vi "Autoscan_MirrorsToSPCM.vi"(6 "Device 4":refnum<k24>, 7 "reference":refnum<vi>, 9 "reference 3":refnum<vi>, 10 "reference 2":refnum<vi>, 11 ".NET Refnum in":refnum<k24>) -> (2 "Device":refnum<k24>, 3 ".NET Refnum out":refnum<k24>)   [LabVIEW 2023]
uses:
  C:/Users/nanometa/Documents/TCSPC_Git_Repo/Source/Thorlabs.MotionControl.FilterFlipperCLI.dll
  Thorlabs.MotionControl.FilterFlipperCLI.dll
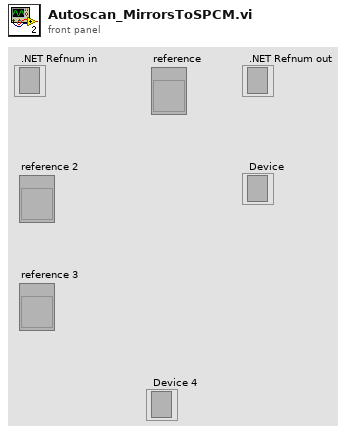
[diagram p1: front panel]
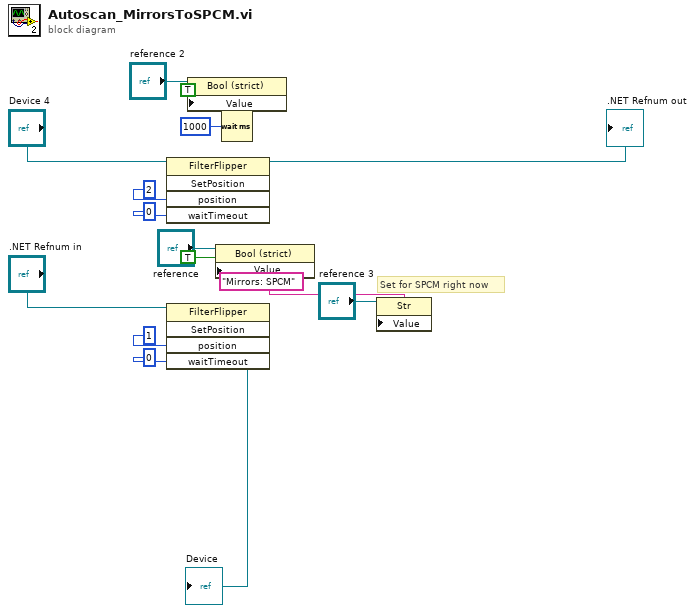
[diagram p0: block diagram]
diagram:
  # "Set for SPCM right now"
  n1 = invoke class="FilterFlipper" method="SetPosition"(reference="Device 4", "position"=u32 2, "waitTimeout"=0) -> (reference out=→".NET Refnum out":refnum<k24>)  [unwired: 2 in, 4 out]
  n2 = invoke class="FilterFlipper" method="SetPosition"(reference=".NET Refnum in", "position"=u32 1, "waitTimeout"=0) -> (reference out=→"Device":refnum<k24>)  [unwired: 2 in, 4 out]
  n3 = property class="Bool (strict)"(reference="reference 2", "Value"=TRUE ("Motion")) -> ()  [unwired: 1 in, 2 out]
  n4 = property class="Bool (strict)"(reference="reference", "Value"=TRUE ("Mirror Movement")) -> ()  [unwired: 1 in, 2 out]
  n5 = Wait (ms)(milliseconds to wait=u32 1000) -> ()  [unwired: 1 out]
  n6 = property class="Str"(reference="reference 3", "Value"="Mirrors: SPCM") -> ()  [unwired: 1 in, 2 out]
